vi "Test Decimation.vi"() -> ()   [LabVIEW 2015]
uses:
  Real-Time/SubVIs/Block descriptor.ctl
  Real-Time/5565/GE5565 Set DMA Transfer Size.vi
  Real-Time/5565/GE5565 Write (U64) Cluster.vi
  Real-Time/SubVIs/Decimation - time to write.vi
  Real-Time/5565/GE5565 Set DMA RW (Cluster) mod.vi
  RefMem DMA Custom Device.lvlib
panel:
  in  "Block descriptors":T1[](array[typedef])=[{"Block Address in Bytes"=0, "Block Decimation \nchannel index"=1, "Transfer size"=0, "FIFO Indexes"=[0, 1, 2], "Channel index in block"=[]}, {"Block Address in Bytes"=0, "Block Decimation \nchannel index"=3, "Transfer size"=0, "FIFO Indexes"=[3, 4, 5], "Channel index in block"=[]}]
  out "Values 2":dbl[](array[numeric])=[1.0, 2.0, 3.0, 4.0, 5.0, 6.0]
  in  "Values":dbl[](array[numeric])=[1.0, 2.0, 3.0, 4.0, 5.0, 6.0]
  in  "stop":bool
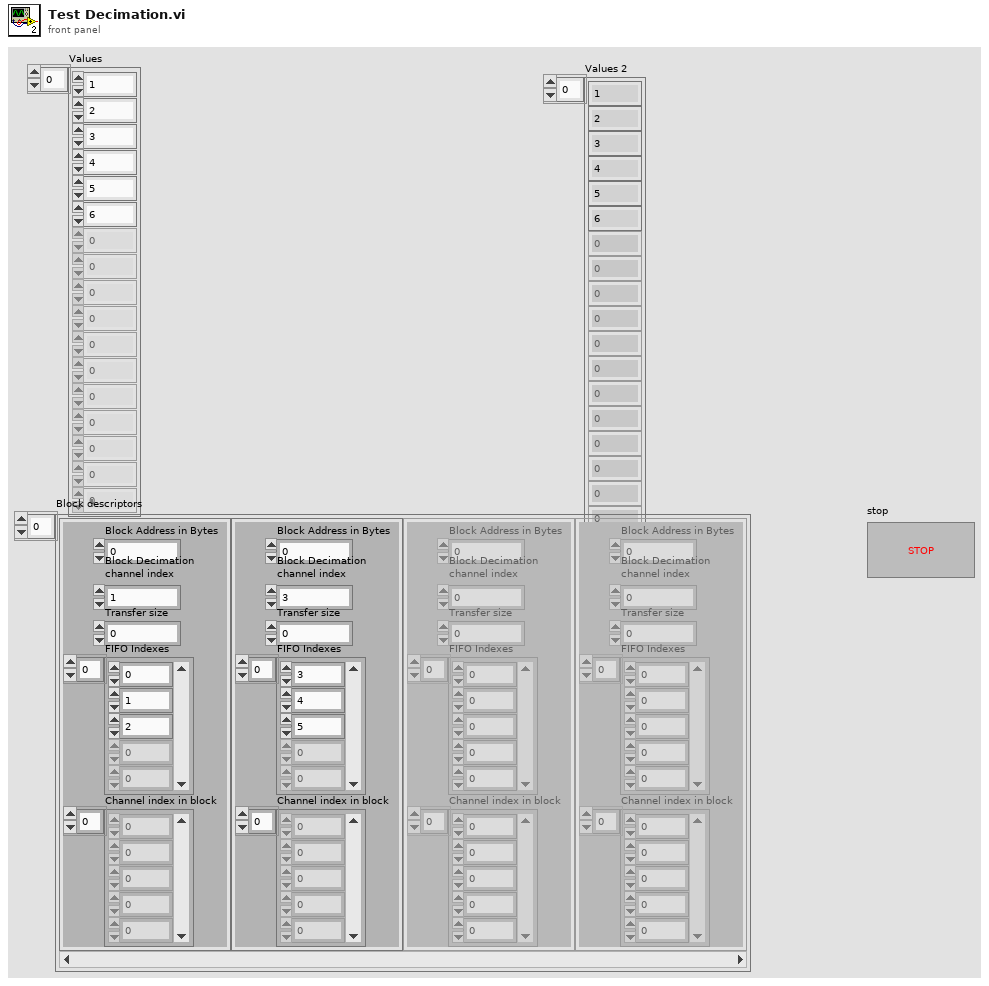
[diagram p1: front panel]
types:
  T1 = typedef "RefMem DMA Custom Device.lvlib/Block descriptor.ctl" = cluster{"Block Address in Bytes":u32, "Block Decimation \nchannel index":i32, "Transfer size":u32, "FIFO Indexes":i32[], "Channel index in block":i32[]}
  T2 = cluster{"VMIC 5565 Resource":refnum<visa-resource-name>, "MEMACC Resource":refnum<visa-resource-name>, "byte count":u32, "mem offset":u32}
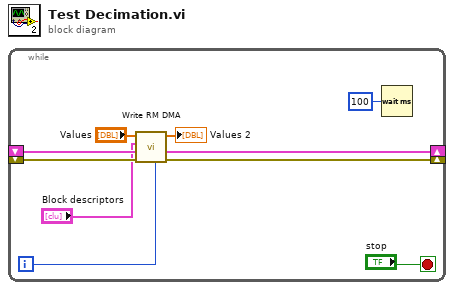
[diagram p0: block diagram]
diagram:
  n1 = while {
    shift-right: [w8] -> _
    shift-left: _ -> [w9]
    shift-right: [w5] -> _
    shift-left: _ -> [w4]
    i -> [w10]
    stop <- "stop" stop-if-true
    n2 = call "Write RM DMA.vi"("Iteration"=w10, "error in"=w9, "VMIC reference in"=w4, "Block descriptors"="Block descriptors", "Values"="Values") -> ("error out"=w8:errorcluster, "VMIC reference out"=w5:T2, "Values"=→"Values 2":dbl[])  [unwired: 3 in, 1 out]
    n3 = Wait (ms)(milliseconds to wait=u32 100) -> ()  [unwired: 1 out]
  }
